vi "Configure Internal Modulation.vi"(0 "VISA resource name":refnum<visa-resource-name>, 1 "Frequency (400 Hz)":dbl=400.0, 2 "Waveform Type (0: Sine)":i32(ring) items=["Sine", "Triangle", "Square", "Ramp", "Pulse", "Noise", "DC"], 5 "Modulation Type (0: Amplitude Modulation)":i32(ring) items=["Amplitude Modulation", "Frequency Modulation", "Phase Modulation", "Low Frequency Output"], 7 "Modulation Path (1: 1)":i32(ring)=1 items=["1"=1, "2"=2], 9 "Tone Path (1: 1)":i32(ring)=1 items=["1"=1, "2"=2], 11 "error in (no error)":errorcluster, 12 "Phase Offset (0 Rad)":dbl, 13 "Ramp Direction (0: Positive)":i32(ring) items=["Positive", "Negative"]) -> (4 "VISA resource name out":refnum<visa-resource-name>, 15 "error out":errorcluster)   [LabVIEW 2012, in "Agilent PSG MXG Series.lvlib"]
doc: "Configures the internal function generator source.\n\n<B>Notes:</B>\n(1) This VI is valid only in N5171B, N5172B, N5181B, N5182B that install <B>Option UNT</B> and <B>Option 303</B> (AM, FM, phase modulation, and LF output)."
uses:
  <instrlib>/Agilent PSG MXG Series/Agilent PSG MXG Series.lvlib
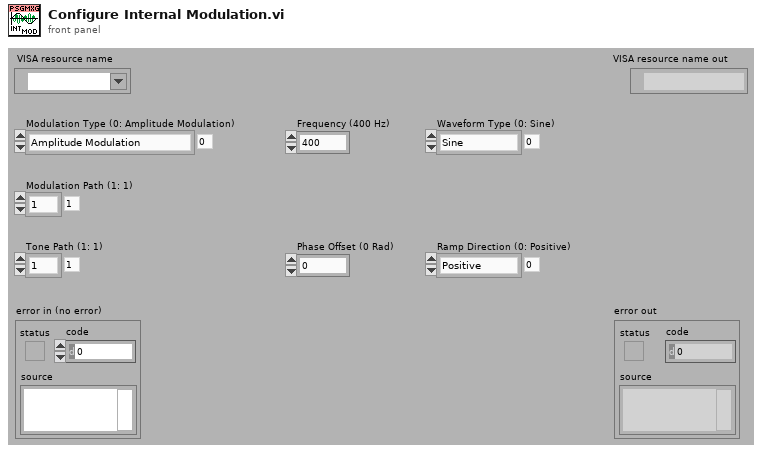
[diagram p1: front panel]
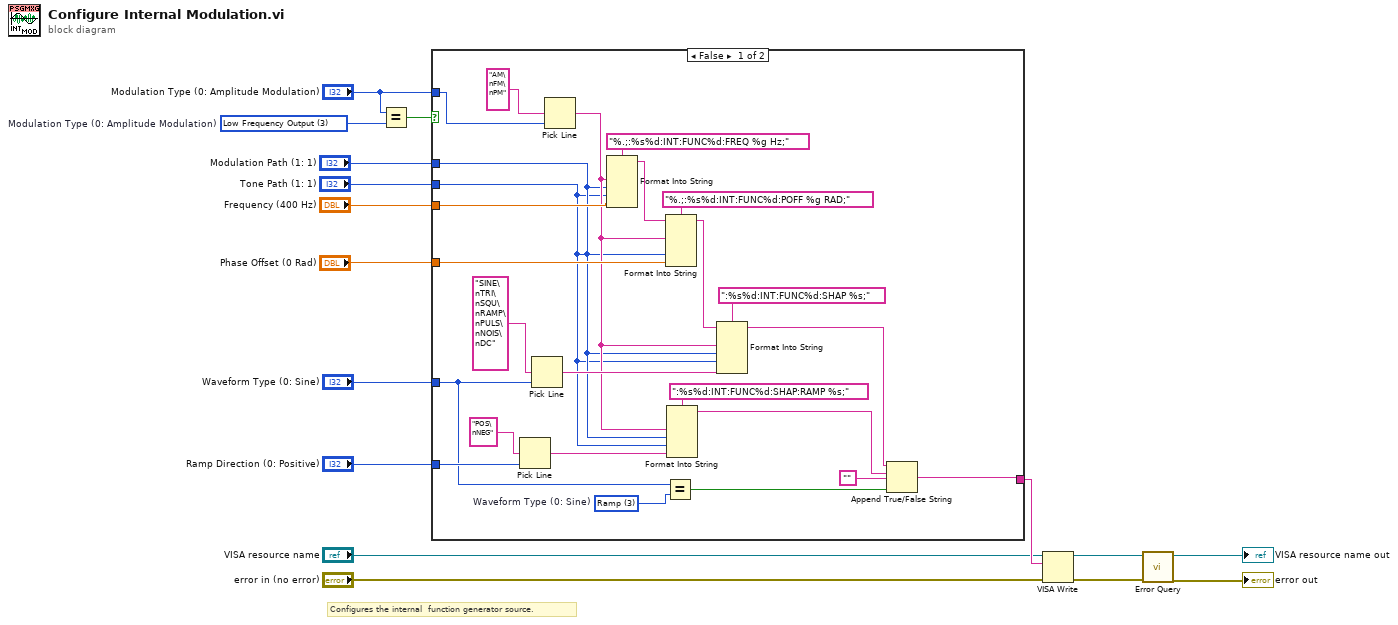
[diagram p0: block diagram]
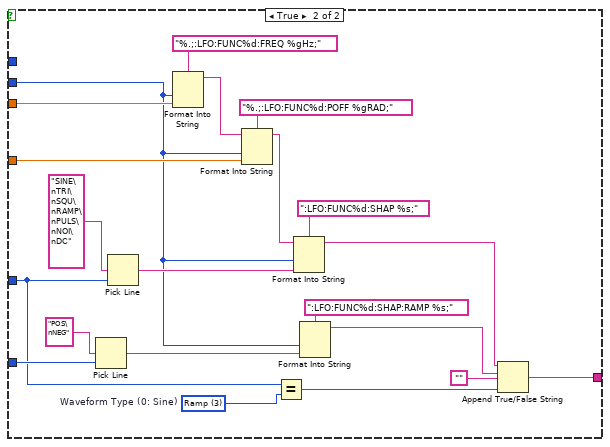
[diagram p2: hidden frame]
diagram:
  w7 = 3 items=["Amplitude Modulation", "Frequency Modulation", "Phase Modulation", "Low Frequency Output"]  # Modulation Type (0: Amplitude Modulation)
  # "Configures the internal  function generator source."
  n1 = Equal?(x="Modulation Type (0: Amplitude Modulation)", y=w7) -> (x = y?=w6:bool)
  n2 = case shown="False" w6 {
    tunnel: "Waveform Type (0: Sine)" -> [w18 w47]
    tunnel: "Ramp Direction (0: Positive)" -> [w34 w51]
    tunnel: [w17 w42] -> w14
    tunnel: "Modulation Type (0: Amplitude Modulation)" -> [w31 _]
    tunnel: "Modulation Path (1: 1)" -> [w26 _]
    tunnel: "Tone Path (1: 1)" -> [w25 w49]
    tunnel: "Frequency (400 Hz)" -> [w30 w54]
    tunnel: "Phase Offset (0 Rad)" -> [w29 w53]
    frame False {
      w21 = 3 items=["Sine", "Triangle", "Square", "Ramp", "Pulse", "Noise", "DC"]  # Waveform Type (0: Sine)
      n3 = Pick Line(multi-line string="POS\nNEG", line index=w34) -> (output string=w24:string)  [unwired: 1 out]
      n4 = Pick Line(multi-line string="SINE\nTRI\nSQU\nRAMP\nPULS\nNOIS\nDC", line index=w18) -> (output string=w28:string)  [unwired: 1 out]
      n5 = Pick Line(multi-line string="AM\nFM\nPM", line index=w31) -> (output string=w27:string)  [unwired: 1 out]
      n6 = Format Into String(format string="%.;:%s%d:INT:FUNC%d:FREQ %g Hz;", w27, w26, w25, w30) -> (resulting string=w40:string)  [unwired: 2 in, 1 out]
      n7 = Equal?(x=w18, y=w21) -> (x = y?=w22:bool)
      n8 = Format Into String(format string="%.;:%s%d:INT:FUNC%d:POFF %g RAD;", initial string=w40, w27, w26, w25, w29) -> (resulting string=w37:string)  [unwired: 1 in, 1 out]
      n9 = Format Into String(format string=":%s%d:INT:FUNC%d:SHAP:RAMP %s;", w27, w26, w25, w24) -> (resulting string=w19:string)  [unwired: 2 in, 1 out]
      n10 = Format Into String(format string=":%s%d:INT:FUNC%d:SHAP %s;", initial string=w37, w27, w26, w25, w28) -> (resulting string=w20:string)  [unwired: 1 in, 1 out]
      n11 = Append True/False String(1:w22, 2:"", 3:w19, 4:w20) -> (0:w17:string)
    }
    frame True {
      w46 = 3 items=["Sine", "Triangle", "Square", "Ramp", "Pulse", "Noise", "DC"]  # Waveform Type (0: Sine)
      n12 = Pick Line(multi-line string="POS\nNEG", line index=w51) -> (output string=w50:string)  [unwired: 1 out]
      n13 = Pick Line(multi-line string="SINE\nTRI\nSQU\nRAMP\nPULS\nNOI\nDC", line index=w47) -> (output string=w52:string)  [unwired: 1 out]
      n14 = Format Into String(format string="%.;:LFO:FUNC%d:FREQ %gHz;", w49, w54) -> (resulting string=w56:string)  [unwired: 2 in, 1 out]
      n15 = Format Into String(format string="%.;:LFO:FUNC%d:POFF %gRAD;", initial string=w56, w49, w53) -> (resulting string=w59:string)  [unwired: 1 in, 1 out]
      n16 = Equal?(x=w47, y=w46) -> (x = y?=w45:bool)
      n17 = Format Into String(format string=":LFO:FUNC%d:SHAP %s;", initial string=w59, w49, w52) -> (resulting string=w48:string)  [unwired: 1 in, 1 out]
      n18 = Format Into String(format string=":LFO:FUNC%d:SHAP:RAMP %s;", w49, w50) -> (resulting string=w43:string)  [unwired: 2 in, 1 out]
      n19 = Append True/False String(1:w45, 2:"", 3:w43, 4:w48) -> (0:w42:string)
    }
  }
  n20 = VISA Write(VISA resource name="VISA resource name", write buffer=w14, error in (no error)="error in (no error)") -> (VISA resource name out=w11:refnum<visa-resource-name>, error out=w10:errorcluster)  [unwired: 1 out]
  n21 = call <instrlib>:"Error Query.vi"("error in (no error)"=w10, "VISA resource name"=w11) -> ("error out"=→"error out":errorcluster, "VISA resource name out"=→"VISA resource name out":refnum<visa-resource-name>)  [unwired: 8 out]
